vi "HexStringToHexDisplayString.vi"(11 "正常显示HEX字符串":string) -> (3 "HEX显示字符串":string)   [LabVIEW 2011]
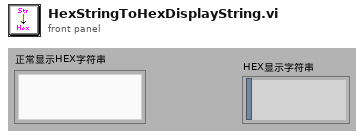
[diagram p1: front panel]
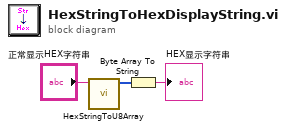
[diagram p0: block diagram]
diagram:
  n1 = call "HexStringToU8Array.vi"("HEX String (0-9,A-F)"="正常显示HEX字符串") -> ("u8 Data[]"=w3:u8[])  [unwired: 10 in]
  n2 = Byte Array To String(unsigned byte array=w3) -> (string=→"HEX显示字符串":string)
